vi "MT Rician Selective Fading profile (Jakes).vi"(0 "profile length (samples)":i32=1000, 1 "rician parameter K (dB)":dbl=2.0 format="%.2f", 2 "number of paths":i32=1, 5 "sampling frequency (Hz)":dbl=1.0 format="%.2f", 7 "doppler spread (Hz)":dbl=0.01 format="%.2p", 9 "seed in (0xFFFFFFFF)":i32=-1 format="%.0x", 11 "error in (no error)":errorcluster, 12 "fading variance":dbl=1.0 format="%.2f", 13 "reset? (T)":bool=TRUE) -> (4 "fading profile":cdb[][](array[numeric]), 10 "seed out":i32 format="%.0x", 15 "error out":errorcluster)   [LabVIEW 2020, in "niDMT.lvlib"]
doc: "This polymorphic instance generates a Rician selective-fading profile for the multipath channel. The envelope for the first path statistically obeys the Rician distribution, while the envelope for the remaining path obeys the Rayleigh distribution implemented using the Jakes model."
uses:
  <vilib>/addons/Modulation/niDMT.lvlib
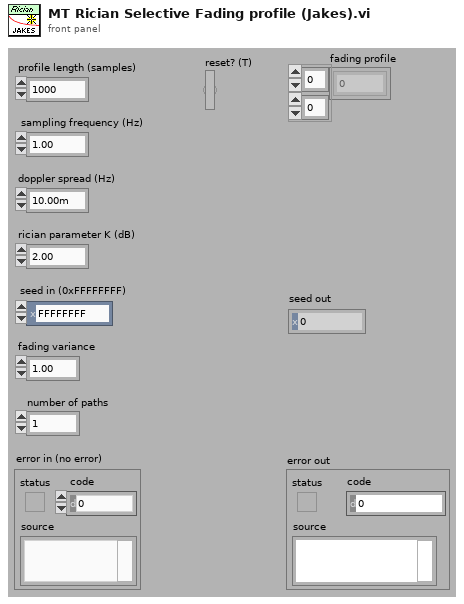
[diagram p1: front panel]
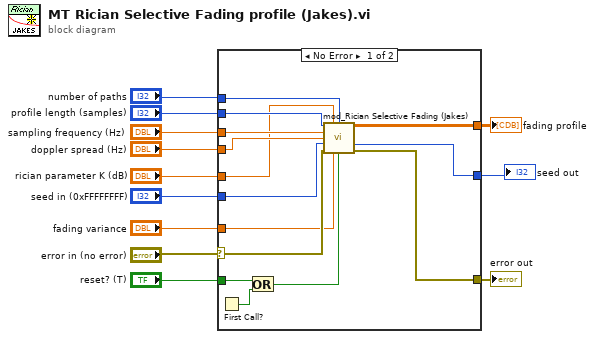
[diagram p0: block diagram]
diagram:
  n1 = case shown="No Error" "error in (no error)" {
    selector: "error in (no error)" -> [w22 w27]
    tunnel: "profile length (samples)" -> [w25 _]
    tunnel: [w26 w27] -> w1
    tunnel: "sampling frequency (Hz)" -> [w24 _]
    tunnel: "doppler spread (Hz)" -> [w23 _]
    tunnel: "reset? (T)" -> [w21 _]
    tunnel: "rician parameter K (dB)" -> [w17 _]
    tunnel: "seed in (0xFFFFFFFF)" -> [w18 _]
    tunnel: "fading variance" -> [w16 _]
    tunnel: [w15 _] -> w4
    tunnel: [w14 _] -> w3
    tunnel: "number of paths" -> [w13 _]
    frame No Error {
      n2 = First Call?() -> (First Call?: T/F=w20:bool)
      n3 = Or(x=w21, y=w20) -> (x .or. y?=w19:bool)
      n4 = call <vilib>:"mod_Rician Selective Fading (Jakes).vi"("profile length (samples)"=w25, "rician parameter K (dB)"=w17, "number of paths"=w13, "sampling frequency (Hz)"=w24, "doppler spread (Hz)"=w23, "seed in (0xFFFFFFFF)"=w18, "error in (no error)"=w22, "fading variance"=w16, "reset? (T)"=w19) -> ("Rician Fading profile"=w14:cdb[][], "next seed"=w15:i32, "error out"=w26:errorcluster)  [unwired: 4 out]
    }
    frame Error {
    }
  }
  "seed out" <- w4
  "fading profile" <- w3
  "error out" <- w1
